vi "edittest import sequence.vi"(6 "User":T2, 8 "error in (no error)":errorcluster, 9 "Content (\"\")":string, 10 "Filename":string, 11 "Connection Refnum":T1) -> (0 "error out":errorcluster, 2 "Sequence Record":T3, 3 "Connection Refnum":T1)   [LabVIEW 2011]
uses:
  server/database/Sequences/Sequence Record.ctl
  server/database/Users/User Record.ctl
  Summitek EXT/ODBC/SQL Controls/Connection Refnum.ctl
  sequence xml.ctl
  server/database/Steps/Step Record.ctl
  server/database/Fields/Field Record.ctl
  server/database/Fields/Field DataTypes.ctl
  server/database/Fields/Field NextItem.ctl
  <vilib>/Utility/config.llb/NI_LVConfig.lvlib
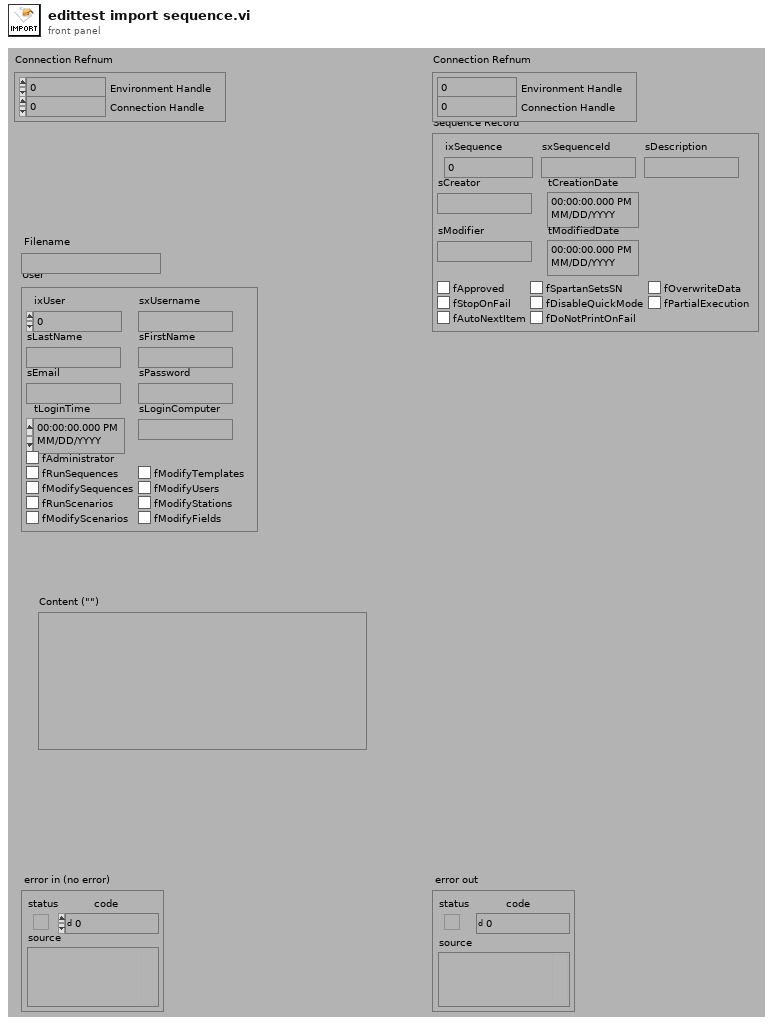
[diagram p1: front panel]
types:
  T1 = typedef "Connection Refnum.ctl" = cluster{"Environment Handle":i32, "Connection Handle":i32}
  T2 = typedef "User Record.ctl" = cluster{"ixUser":i32, "sxUsername":string, "sLastName":string, "sFirstName":string, "sEmail":string, "sPassword":string, "tLoginTime":timestamp, "sLoginComputer":string, "fAdministrator":bool, "fRunSequences":bool, "fModifySequences":bool, "fRunScenarios":bool, "fModifyScenarios":bool, "fModifyTemplates":bool, "fModifyUsers":bool, "fModifyStations":bool, "fModifyFields":bool}
  T3 = typedef "Sequence Record.ctl" = cluster{"ixSequence":i32, "sxSequenceId":string, "sDescription":string, "sCreator":string, "tCreationDate":timestamp, "sModifier":string, "tModifiedDate":timestamp, "fApproved":bool, "fSpartanSetsSN":bool, "fOverwriteData":bool, "fStopOnFail":bool, "fDisableQuickMode":bool, "fPartialExecution":bool, "fAutoNextItem":bool, "fDoNotPrintOnFail":bool}
  T4 = typedef "sequence xml.ctl" = cluster{"#attributes":cluster{"Version":string, "Creator":string}, "Sequence":T3, "Steps":T5[], "Fields":T6[]}
  T5 = typedef "Step Record.ctl" = cluster{"ixStep":i32, "sxSequenceId":string, "sxTestId":string, "iIndex":i32, "iRepeat":i32, "iQuickMode":i32, "sTag":string, "sDatasheetsCSV":string, "bConfiguration":string}
  T6 = typedef "Field Record.ctl" = cluster{"ixField":i32, "iSequenceOrder":i32, "sxFieldId":string, "sxSequenceId":string, "sDisplayName":string, "sValue":string, "sUnits":string, "nDataType":T7, "nNextItem":T8, "fSystem":bool, "fSystemValue":bool, "fRequired":bool, "fSetAtTest":bool, "fTestField":bool, "fDeleted":bool, "fIndexed":bool, "fFreeList":bool}
  T7 = typedef "Field DataTypes.ctl" = enum32{"text", "numeric", "list", "timestamp", "boolean"}
  T8 = typedef "Field NextItem.ctl" = enum32{"Reset", "Retain", "Auto-Increment"}
  T9 = typedef "NI_LVConfig.lvlib/Config Data RefNum.ctl" = refnum<k1>
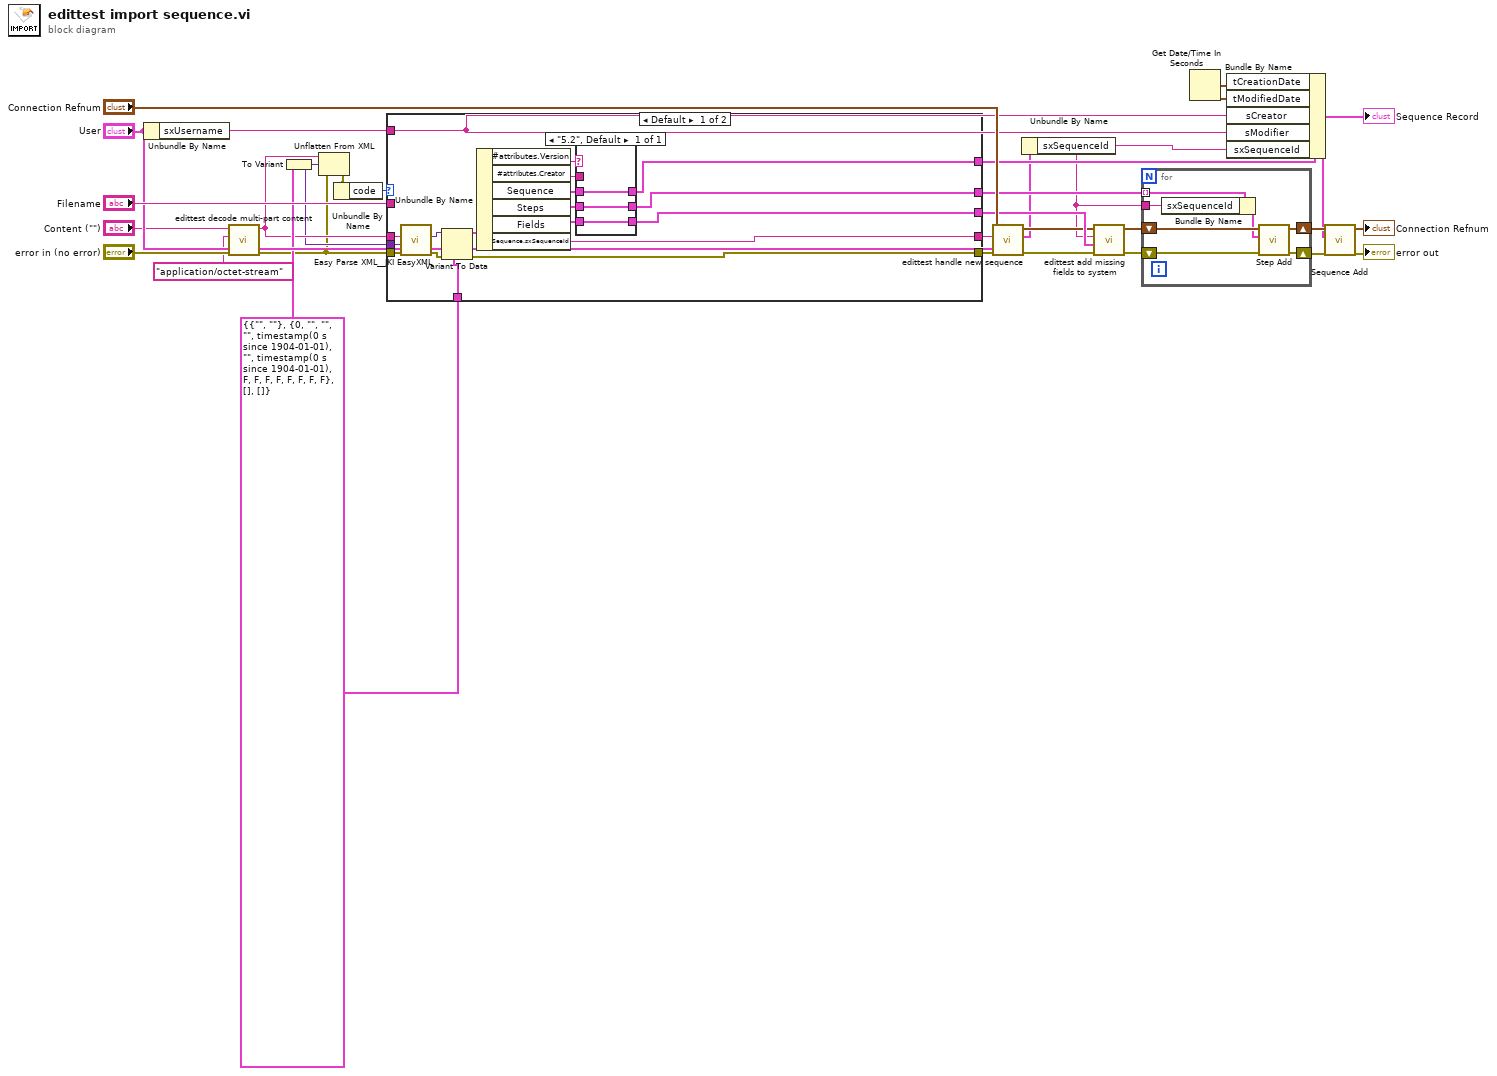
[diagram p0: block diagram]
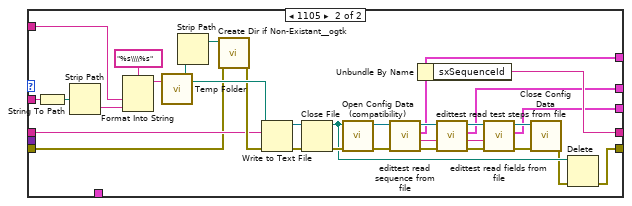
[diagram p2: hidden frame]
diagram:
  w4 = T4 {"#attributes"={"Version"="", "Creator"=""}, "Sequence"={"ixSequence"=0, "sxSequenceId"="", "sDescription"="", "sCreator"="", "tCreationDate"=timestamp(0 s since 1904-01-01), "sModifier"="", "tModifiedDate"=timestamp(0 s since 1904-01-01), "fApproved"=FALSE, "fSpartanSetsSN"=FALSE, "fOverwriteData"=FALSE, "fStopOnFail"=FALSE, "fDisableQuickMode"=FALSE, "fPartialExecution"=FALSE, "fAutoNextItem"=FALSE, "fDoNotPrintOnFail"=FALSE}, "Steps"=[], "Fields"=[]} ("Sequence")
  n1 = Unbundle By Name("User") -> ("sxUsername"=w23:string)
  n2 = call "edittest decode multi-part content.vi"("error in (no error)"="error in (no error)", "Valid Content-Type: (\"text/xml\")"="application/octet-stream" ("Relative Path (\"\" - Folder)"), "Multi-Part Content (\"\")"="Content (\"\")") -> ("error out"=w1:errorcluster, "Content"=w3:string)  [unwired: 7 out]
  n3 = To Variant(anything=w4) -> (Variant=w2:variant)
  n4 = Unflatten From XML(xml string=w3, type=w2, error in (no error)=w1) -> (error out=w5:errorcluster)  [unwired: 1 out]
  n5 = Unbundle By Name(w5) -> ("code"=w6:i32)
  n6 = case shown="Default" w6 {
    tunnel: [w33 w63] -> w29
    tunnel: [w36 w62] -> w28
    tunnel: "Filename" -> [_ w60]
    tunnel: [w45 w56] -> w26
    tunnel: [w34 w55] -> w24
    tunnel: w23 -> [_ w54]
    tunnel: [w35 w53] -> w20
    tunnel: w1 -> [w44 w51]
    tunnel: w3 -> [w43 w52]
    tunnel: w2 -> [w32 _]
    tunnel: w4 -> [w31 _]
    frame Default {
      n7 = call "Easy Parse XML__JKI EasyXML.vi"("error in (no error)"=w44, "LabVIEW Data (Type)"=w32, "XML String"=w43) -> ("error out"=w47:errorcluster, "LabVIEW Data"=w46:variant)  [unwired: 7 out]
      n8 = Variant To Data(error in=w47, type=w31, Variant=w46) -> (data=w42:T4, error out=w45:errorcluster)
      n9 = Unbundle By Name(w42) -> ("#attributes.Version"=w41:string, "#attributes.Creator"=w40:string, "Sequence"=w39:T3, "Steps"=w38:T5[], "Fields"=w37:T6[], "Sequence.sxSequenceId"=w33:string)
      n10 = case shown="\"5.2\", Default" w41 {
        tunnel: w40 -> [_]
        tunnel: w39 -> [w50]
        tunnel: w38 -> [w49]
        tunnel: w37 -> [w48]
        tunnel: [w50] -> w36
        tunnel: [w49] -> w35
        tunnel: [w48] -> w34
        frame "5.2", Default {
        }
      }
    }
    frame 1105 {
      n11 = String To Path(string=w60) -> (path=w61:path)
      n12 = Strip Path(path=w61) -> (name=w59:string)  [unwired: 1 out]
      n13 = Format Into String(format string="%s\\\\%s" ("Relative Path (\"\" - Folder)"), w54, w59) -> (resulting string=w68:string)  [unwired: 2 in, 1 out]
      n14 = call "Temp Folder.vi"("Relative Path (\"\")"=w68) -> ("Temp Folder"=w65:path)  [unwired: 2 out]
      n15 = Strip Path(path=w65) -> (stripped path=w66:path)  [unwired: 1 out]
      n16 = call "Create Dir if Non-Existant__ogtk.vi"("error in (no error)"=w51, "Directory Path"=w66) -> ("error out"=w64:errorcluster)  [unwired: 1 in, 8 out]
      n17 = Write to Text File(file (use dialog)=w65, text=w52, error in=w64) -> (refnum out=w70:refnum<file>, error out=w72:errorcluster)  [unwired: 2 out]
      n18 = Close File(refnum=w70, error in=w72) -> (path=w58:path, error out=w71:errorcluster)
      n19 = call <vilib>:"Open Config Data (compatibility).vi"("error in (no error)"=w71, "configuration file path"=w58) -> ("error out"=w80:errorcluster, "refnum"=w67:T9)  [unwired: 7 in, 1 out]
      n20 = call "edittest read sequence from file.vi"("error in (no error)"=w80, "File Refnum In"=w67) -> ("error out"=w79:errorcluster, "Version"=w73:string, "Sequence Record"=w62:T3, "File Refnum Out"=w78:T9)  [unwired: 6 out]
      n21 = Unbundle By Name(w62) -> ("sxSequenceId"=w63:string)
      n22 = call "edittest read test steps from file.vi"("error in (no error)"=w79, "Version"=w73, "File Refnum In"=w78) -> ("error out"=w77:errorcluster, "Sequence Steps"=w53:T5[], "File Refnum Out"=w76:T9)  [unwired: 6 out]
      n23 = call "edittest read fields from file.vi"("error in (no error)"=w77, "Version"=w73, "File Refnum In"=w76) -> ("error out"=w74:errorcluster, "Sequence Fields"=w55:T6[], "File Refnum Out"=w75:T9)  [unwired: 6 out]
      n24 = call <vilib>:"Close Config Data.vi"("error in (no error)"=w74, "refnum"=w75) -> ("error out"=w57:errorcluster)  [unwired: 1 in, 8 out]
      n25 = Delete(path (use dialog)=w58, error in=w57) -> (error out=w56:errorcluster)  [unwired: 5 out]
    }
  }
  n26 = call "edittest handle new sequence.vi"("User Information"="User", "error in (no error)"=w26, "New Name Suggestion\n(empty - \"Username Sequence N\")"=w29, "Connection Refnum"="Connection Refnum") -> ("error out"=w25:errorcluster, "New Sequence Record"=w16:T3, "Connection Refnum"=w17:T1)  [unwired: 5 out]
  n27 = Unbundle By Name(w16) -> ("sxSequenceId"=w10:string)
  n28 = call "edittest add missing fields to system.vi"("error in (no error)"=w25, "Fields"=w24, "sxSequenceId (\"\")"=w10, "Connection Refnum"=w17) -> ("error out"=w18:errorcluster, "Connection Refnum"=w19:T1)  [unwired: 6 out]
  n29 = for {
    tunnel: w20 -> [w83] mode=indexing
    shift-right: [w84] -> w15
    shift-left: w18 -> [w86]
    shift-right: [w85] -> w13
    shift-left: w19 -> [w87]
    tunnel: w10 -> [w82]
    n30 = Bundle By Name(cluster=w83, "sxSequenceId"=w82) -> (w81:T5)
    n31 = call "Step Add.vi"("error in (no error)"=w86, "Step Record"=w81, "Connection Refnum"=w87) -> ("error out"=w84:errorcluster, "Connection Refnum"=w85:T1)  [unwired: 7 out]
  }
  n32 = Get Date/Time In Seconds() -> (seconds since 1Jan1904=w22:timestamp)
  n33 = Bundle By Name(cluster=w28, "tCreationDate"=w22, "tModifiedDate"=w22, "sCreator"=w23, "sModifier"=w23, "sxSequenceId"=w10) -> (w11:T3)
  "Sequence Record" <- w11
  n34 = call "Sequence Add.vi"("error in (no error)"=w15, "Sequence Record"=w11, "Connection Refnum"=w13) -> ("error out"=→"error out":errorcluster, "Connection Refnum"=→"Connection Refnum":T1)  [unwired: 7 out]
